vi "Keyance Setup.vi"(8 "error in":errorcluster, 11 "Laser Etcher In":refnum<visa-resource-name>) -> (0 "error out":errorcluster, 3 "Laser Etcher Out":refnum<visa-resource-name>)   [LabVIEW 2023]
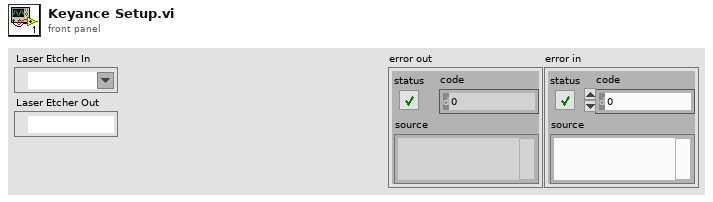
[diagram p1: front panel]
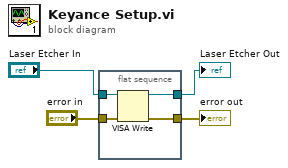
[diagram p0: block diagram]
diagram:
  n1 = flat-sequence {
    tunnel: [w5] -> w4
    tunnel: [w6] -> w3
    tunnel: "error in" -> [w8]
    tunnel: "Laser Etcher In" -> [w7]
    frame #0 {
      n2 = VISA Write(VISA resource name=w7, error in (no error)=w8) -> (VISA resource name out=w6:refnum<visa-resource-name>, error out=w5:errorcluster)  [unwired: 1 in, 1 out]
    }
  }
  "Laser Etcher Out" <- w3
  "error out" <- w4
